vi "Timestamp String to LV Timestamp Array.vi"(0 "Array":string[](array[string])) -> (1 "Y M D H M S Array":i32[][](array[numeric]), 2 "Array 2":timestamp[](array[timestamp]))   [LabVIEW 2018]
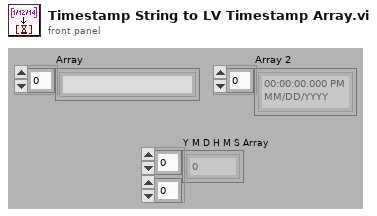
[diagram p1: front panel]
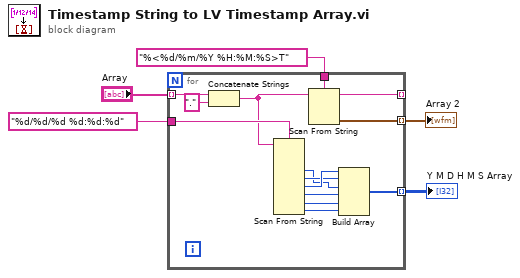
[diagram p0: block diagram]
diagram:
  n1 = for {
    tunnel: "%<%d/%m/%Y %H:%M:%S>T" ("format string") -> [w19]
    tunnel: "Array" -> [w16] mode=indexing
    tunnel: [w18] -> w4 mode=indexing
    tunnel: [w17] -> _ mode=indexing
    tunnel: "%d/%d/%d %d:%d:%d" ("format string") -> [w8]
    tunnel: [w7] -> w1 mode=indexing
    n2 = Concatenate Strings(w16, "." ("string")) -> (w6:string)
    n3 = Scan From String(format string=w8, input string=w6) -> (output 1=w12:i32, output 2=w13:i32, output 3=w14:i32, output 4=w11:i32, output 5=w10:i32, output 6=w9:i32)  [unwired: 8 in, 3 out]
    n4 = Scan From String(format string=w19, input string=w6) -> (remaining string=w17:string, output 1=w18:timestamp)  [unwired: 3 in, 2 out]
    n5 = Build Array(w14, w13, w12, w11, w10, w9) -> (w7:i32[])
  }
  "Array 2" <- w4
  "Y M D H M S Array" <- w1
